vi "GUI - Text File (V1.00).vi"(0 "Time Data IN":refnum<class "GSwFormDSP.lvclass">, 5 "error in (no error)":errorcluster, 6 "Inlude Time Vector":bool, 7 "Application Name":string="GSwForm", 9 "State Queue":string[](array[string])=["SC: Initialize"], 11 "TextFile - READ":path, 13 "TextFile - WRITE":path) -> (14 "Time Data DUP":refnum<class "GSwFormDSP.lvclass">, 19 "error out":errorcluster)   [LabVIEW 2022 SP3, in "TEXT.lvclass"]
uses:
  TEXT.lvclass
  API/GSwFormDSP_class/GSwFormDSP.lvclass
  <vilib>/Utility/sysdir.llb/System Directory Type.ctl
  W:/projects/archives/23 Charette AI Group/SPWB/API/Generic Utilities_class/Generic Utilities.lvclass
  <vilib>/addons/_AddQ/G#Object/G#Object.lvclass
  API/Generic Utilities_class/Generic Utilities.lvclass
panel:
  in  "Task":enum32{"TDMS", "Settings"}(tab)
  out "Time Data":waveform(dbl)[](graph)
  in  "READ - Select Wave File":bool
  in  "WRITE - Select Wave File":bool
  out "State History":string[](array[string])
  out "State Index":i32
  in  "Exit":bool
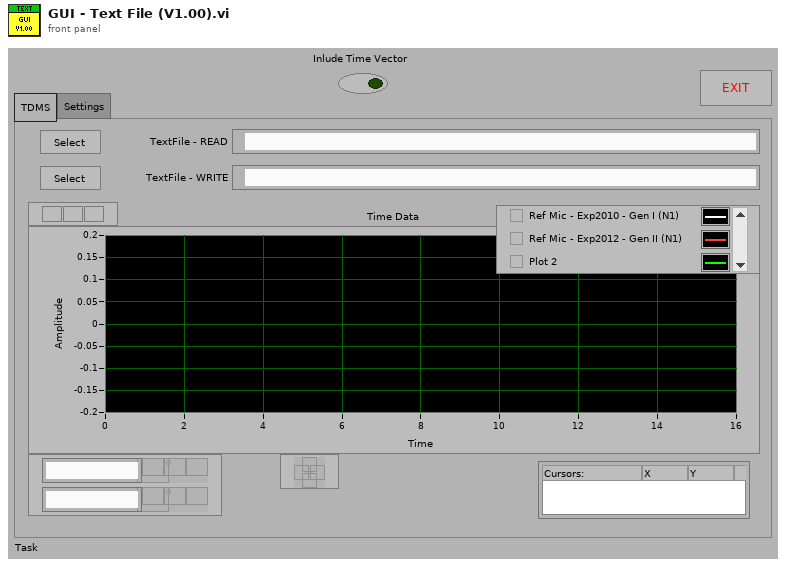
[diagram p1: front panel]
types:
  T1 = enum32{"Invalid", "Standard", "Closed", "Hidden", "Minimized", "Maximized"}
  T2 = typedef "System Directory Type.ctl" = i32
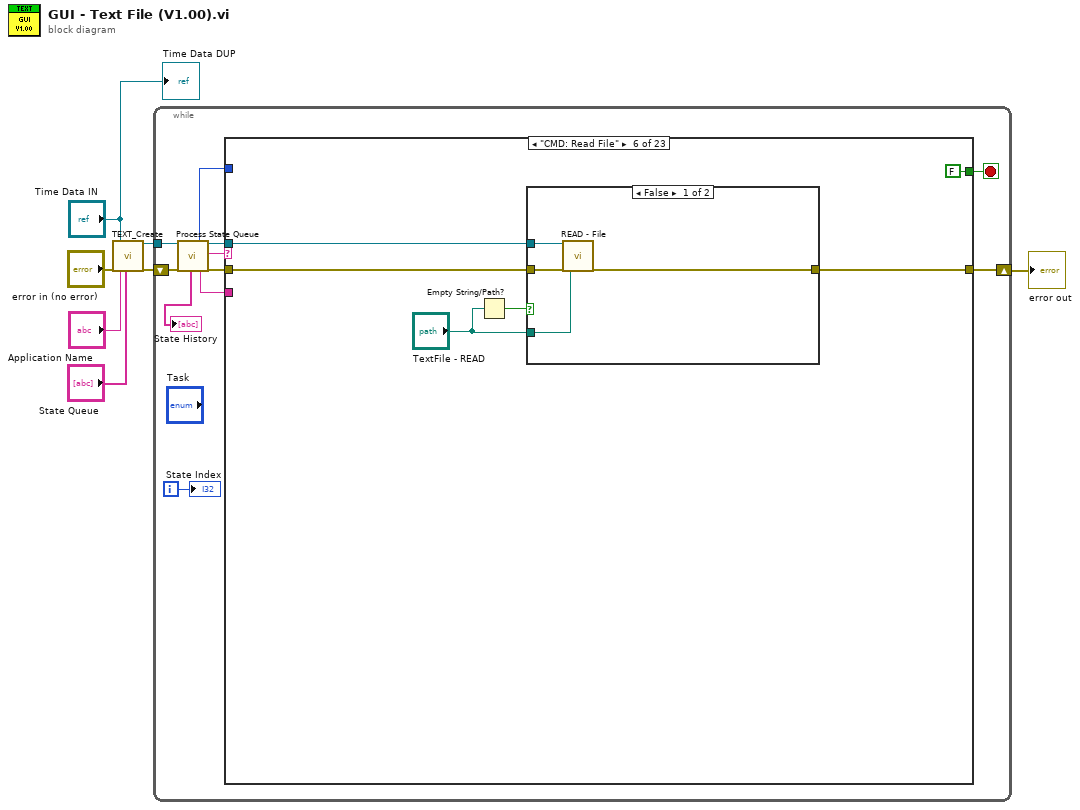
[diagram p0: block diagram]
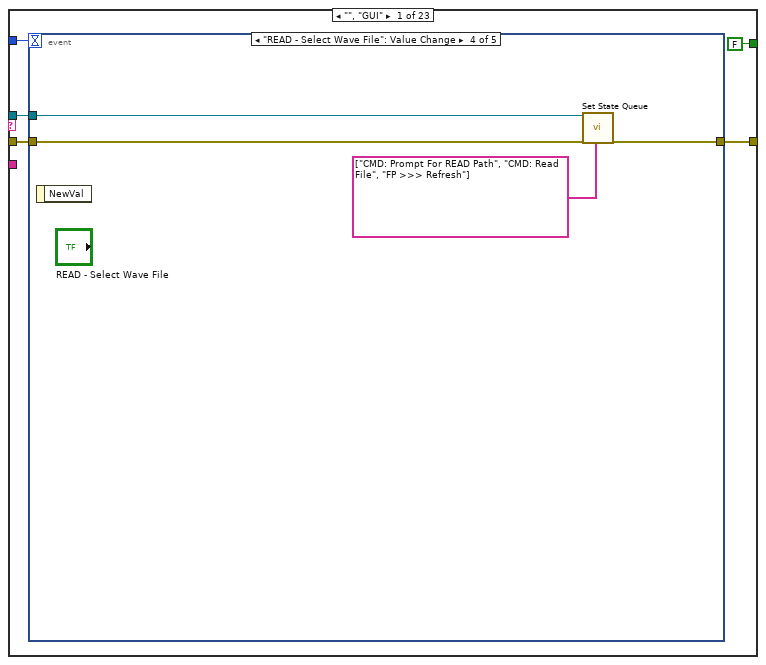
[diagram p2: hidden frame]
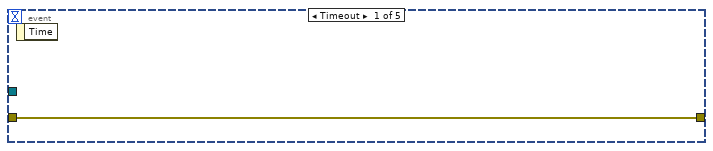
[diagram p3: hidden frame]
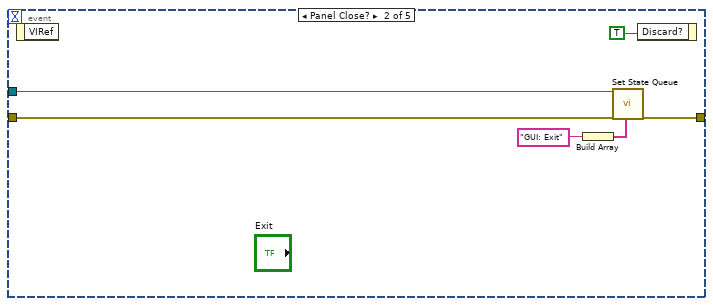
[diagram p4: hidden frame]
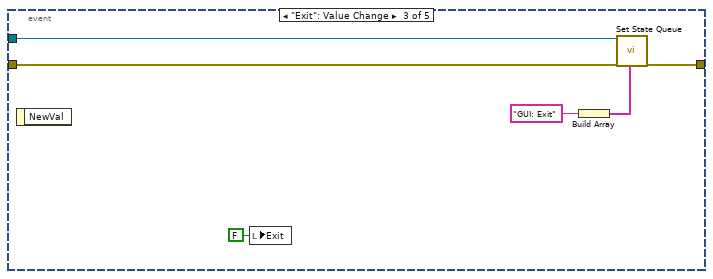
[diagram p5: hidden frame]
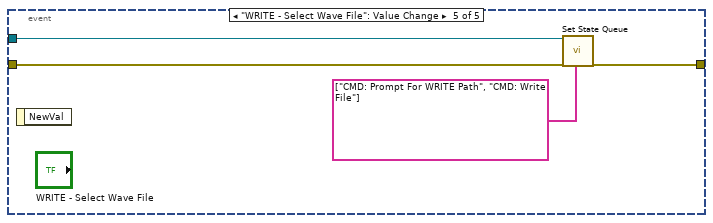
[diagram p6: hidden frame]
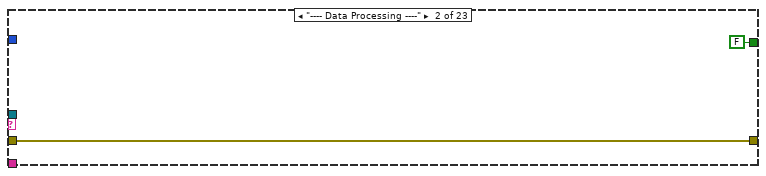
[diagram p7: hidden frame]
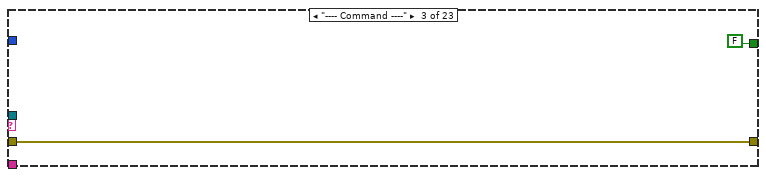
[diagram p8: hidden frame]
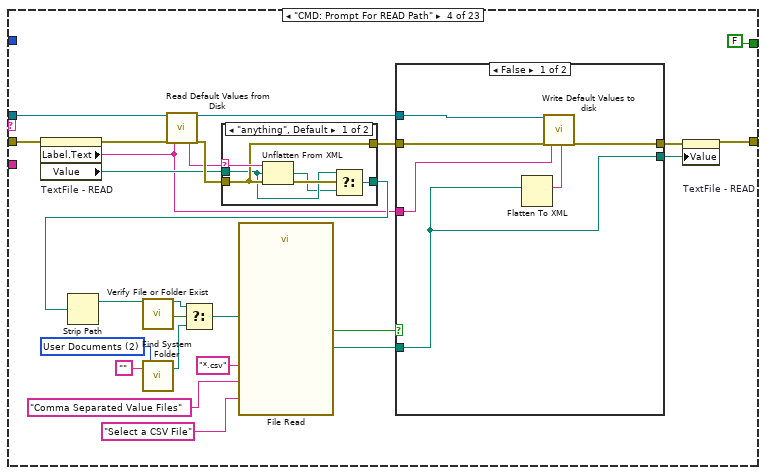
[diagram p9: hidden frame]
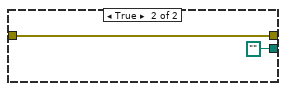
[diagram p10: hidden frame]
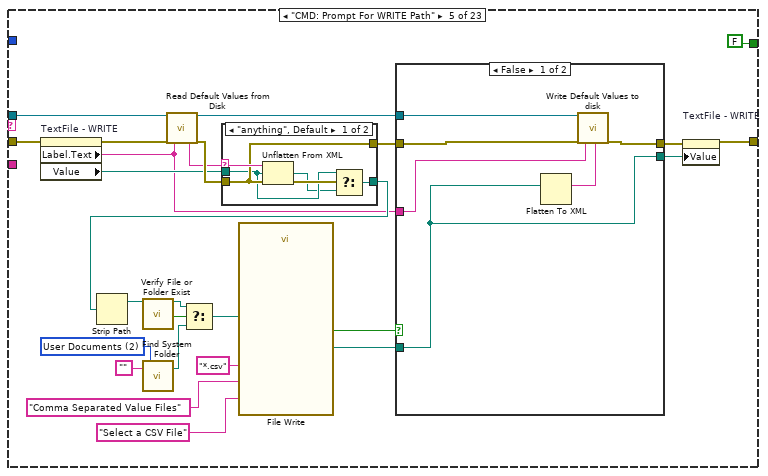
[diagram p12: hidden frame]
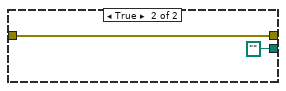
[diagram p13: hidden frame]
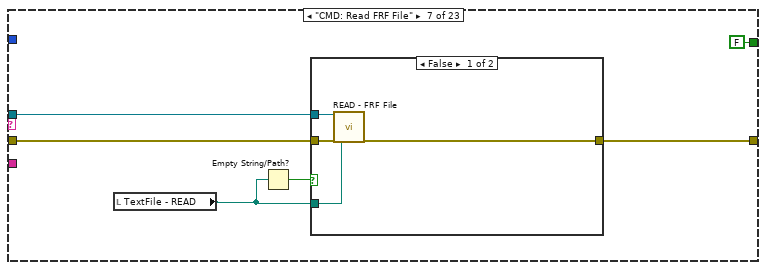
[diagram p16: hidden frame]
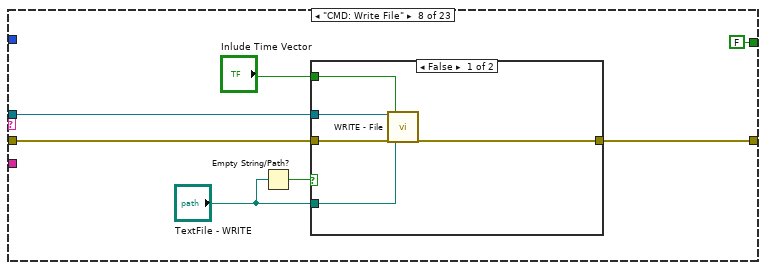
[diagram p18: hidden frame]
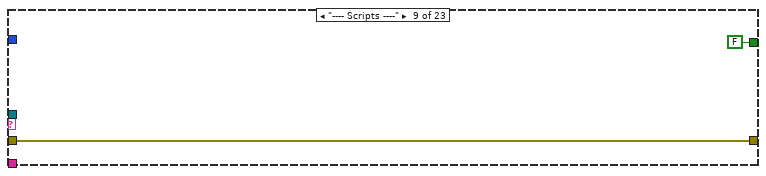
[diagram p20: hidden frame]
diagram:
  n1 = call "TEXT_Create.vi"("error in (no error)"="error in (no error)", "Time Data"="Time Data IN", "Application Name"="Application Name", "State Queue"="State Queue") -> ("reference out"=w7:refnum<class "TEXT.lvclass">, "error out"=w6:errorcluster)  [unwired: 14 in]
  n2 = while {
    shift-right: [w9] -> w2
    shift-left: w6 -> [w15]
    tunnel: w7 -> [w16]
    i -> [w17]
    stop <- w18 stop-if-true
    n3 = call "Process State Queue.vi"("reference in"=w16, "error in (no error)"=w15) -> ("State History"=→"State History":string[], "Timeout"=w14:i32, "State Option"=w11:string, "reference out"=w13:refnum<class "TEXT.lvclass">, "Current State"=w12:string, "error out"=w10:errorcluster)  [unwired: 10 in, 2 out]
    n4 = case shown="\"CMD: Read File\"" w12 {
      selector: w12 -> [_ _ _ _ _ _ _ _ _ _ _ _ _ _ _ _ _ _ _ w344 _ _ _]
      tunnel: w13 -> [w21 _ _ w73 w115 w137 w148 w160 _ w173 _ w179 w209 _ w249 w268 w301 w326 _ _ _ _ w352]
      tunnel: [FALSE FALSE FALSE FALSE FALSE FALSE FALSE FALSE FALSE FALSE FALSE FALSE FALSE FALSE FALSE TRUE FALSE FALSE FALSE FALSE FALSE FALSE TRUE] -> w18
      tunnel: w14 -> [w22 _ _ _ _ _ _ _ _ _ _ _ _ _ _ _ _ _ _ _ _ _ _]
      tunnel: w11 -> [_ _ _ _ _ _ _ _ _ _ _ w180 w206 _ _ _ w310 _ _ _ _ _ _]
      tunnel: w10 -> [w20 w45 w47 w72 w114 w136 w147 w159 w168 w172 w175 w177 w208 w235 w246 w265 w300 w327 w340 w342 w347 w350 w353]
      tunnel: [w19 w45 w47 w56 w100 w135 w146 w158 w168 w171 w175 w178 w207 w235 w237 w264 w298 w323 w340 w342 errorcluster {"status"=FALSE, "code"=0, "source"=""} ("error out") w350 w354] -> w9
      frame "", "GUI" {
        n5 = event shown="[3] \"READ - Select Wave File\": Value Change" {
          selector: _ -> [_ _ _ _ _]
          dyn-events: _ -> [_ _ _ _ _]
          timeout: w22 -> [_ _ _ _ _]
          tunnel: w21 -> [_ w28 w34 w39 w43]
          tunnel: w20 -> [w24 w27 w32 w38 w42]
          tunnel: [w24 w26 w33 w40 w44] -> w19
          event Timeout {
            n6 = event-data() -> ()  [unwired: 1 in, 1 out]
          }
          event Panel Close? {
            n7 = event-data() -> ()  [unwired: 1 in, 1 out]
            n8 = Build Array("GUI: Exit") -> (w25:string[])
            n9 = call "Set State Queue.vi"("reference in"=w28, "error in (no error)"=w27, "State Queue"=w25) -> ("error out"=w26:errorcluster)  [unwired: 15 in, 1 out]
            n10 = event-data("Discard?"=TRUE) -> ()  [unwired: 1 in, 1 out]
          }
          event "Exit": Value Change {
            n11 = event-data() -> ()  [unwired: 1 in, 1 out]
            n12 = local write "Exit"(FALSE ("Exit")) -> ()
            n13 = Build Array("GUI: Exit") -> (w31:string[])
            n14 = call "Set State Queue.vi"("reference in"=w34, "error in (no error)"=w32, "State Queue"=w31) -> ("error out"=w33:errorcluster)  [unwired: 15 in, 1 out]
          }
          event "READ - Select Wave File": Value Change {
            n15 = event-data() -> ()  [unwired: 1 in, 1 out]
            n16 = call "Set State Queue.vi"("reference in"=w39, "error in (no error)"=w38, "State Queue"=string[] ["CMD: Prompt For READ Path", "CMD: Read File", "FP >>> Refresh"]) -> ("error out"=w40:errorcluster)  [unwired: 15 in, 1 out]
          }
          event "WRITE - Select Wave File": Value Change {
            n17 = event-data() -> ()  [unwired: 1 in, 1 out]
            n18 = call "Set State Queue.vi"("reference in"=w43, "error in (no error)"=w42, "State Queue"=string[] ["CMD: Prompt For WRITE Path", "CMD: Write File"]) -> ("error out"=w44:errorcluster)  [unwired: 15 in, 1 out]
          }
        }
      }
      frame "---- Data Processing ----" {
      }
      frame "---- Command ----" {
      }
      frame "CMD: Prompt For READ Path" {
        w63 = T2 2 items=["User Home"=0, "User Desktop"=1, "User Documents"=2, "User Application Data"=3, "User Preferences"=4, "User Temporary"=5, "Public Documents"=6, "Public Application Data"=7, "Public Preferences"=8, "Public Cache"=13, "System Core Libraries"=9, "System Installed Libraries"=10, "Application Files"=11, "Boot Volume Root"=12] ("system directory type")
        n19 = property on="TextFile - READ" class="Path"(error in=w72) -> (error out=w71:errorcluster, "Label.Text"=w51:string, "Value"=w69:path)  [unwired: 1 in, 1 out]
        n20 = call "Find System Folder.vi"("Application Name"="", "system directory type"=w63) -> ("System Folder"=w62:path)  [unwired: 16 in, 1 out]
        n21 = call-dynamic "Read Default Values from Disk.vi"("reference in"=w73, "error in (no error)"=w71, "Control Label"=w51) -> ("Value (XML String)"=w49:string, "reference out"=w52:refnum<class "TEXT.lvclass">, "error out"=w70:errorcluster)  [unwired: 14 in]
        n22 = case shown="\"anything\", Default" w49 {
          selector: w49 -> [w88 _]
          tunnel: [w83 w90] -> w68
          tunnel: w69 -> [w85 w90]
          tunnel: w70 -> [w86 w89]
          tunnel: [w86 w89] -> w54
          frame "anything", Default {
            n23 = Unflatten From XML(xml string=w88, type=w85, error in (no error)=w86) -> (value=w84:path, error out=w87:errorcluster)
            n24 = Select(t=w85, s=w87, f=w84) -> (s? t:f=w83:path)
          }
          frame "" {
            # "Either the file was not found or there was some error"
          }
        }
        n25 = Strip Path(path=w68) -> (stripped path=w67:path)  [unwired: 1 out]
        n26 = call "Verify File or Folder Exist.vi"("path"=w67) -> ("dup path"=w65:path, "file or folder exists?"=w66:bool)  [unwired: 16 in, 1 out]
        n27 = Select(t=w65, s=w66, f=w62) -> (s? t:f=w64:path)
        n28 = call "File Read"("start path"=w64, "button label"="Select a CSV File", "pattern (all files)"="*.csv", "pattern label"="Comma Separated Value Files") -> ("selected path"=w50:path, "cancelled"=w57:bool)  [unwired: 8 in, 2 out]
        n29 = case shown="False" w57 {
          tunnel: [w76 w82] -> w55
          tunnel: w54 -> [w77 w82]
          tunnel: [w75 path ""] -> w53
          tunnel: w52 -> [w79 _]
          tunnel: w51 -> [w78 _]
          tunnel: w50 -> [w75 _]
          frame False {
            n30 = Flatten To XML(6:w75) -> (2:w80:string)
            n31 = call-dynamic "Write Default Values to disk.vi"("reference in"=w79, "error in (no error)"=w77, "Control Label"=w78, "Value (XML String)"=w80) -> ("error out"=w76:errorcluster)  [unwired: 14 in, 1 out]
          }
          frame True {
          }
        }
        n32 = property on="TextFile - READ" class="Path"(error in=w55, "Value"=w53) -> (error out=w56:errorcluster)  [unwired: 1 in, 1 out]
      }
      frame "CMD: Prompt For WRITE Path" {
        w105 = T2 2 items=["User Home"=0, "User Desktop"=1, "User Documents"=2, "User Application Data"=3, "User Preferences"=4, "User Temporary"=5, "Public Documents"=6, "Public Application Data"=7, "Public Preferences"=8, "Public Cache"=13, "System Core Libraries"=9, "System Installed Libraries"=10, "Application Files"=11, "Boot Volume Root"=12] ("system directory type")
        n33 = property on="TextFile - WRITE" class="Path"(error in=w114) -> (error out=w113:errorcluster, "Label.Text"=w95:string, "Value"=w111:path)  [unwired: 1 in, 1 out]
        n34 = call "Find System Folder.vi"("Application Name"="", "system directory type"=w105) -> ("System Folder"=w104:path)  [unwired: 16 in, 1 out]
        n35 = call-dynamic "Read Default Values from Disk.vi"("reference in"=w115, "error in (no error)"=w113, "Control Label"=w95) -> ("Value (XML String)"=w91:string, "reference out"=w96:refnum<class "TEXT.lvclass">, "error out"=w112:errorcluster)  [unwired: 14 in]
        n36 = case shown="\"anything\", Default" w91 {
          selector: w91 -> [w130 _]
          tunnel: [w125 w132] -> w110
          tunnel: w111 -> [w127 w132]
          tunnel: w112 -> [w128 w131]
          tunnel: [w128 w131] -> w98
          frame "anything", Default {
            n37 = Unflatten From XML(xml string=w130, type=w127, error in (no error)=w128) -> (value=w126:path, error out=w129:errorcluster)
            n38 = Select(t=w127, s=w129, f=w126) -> (s? t:f=w125:path)
          }
          frame "" {
            # "Either the file was not found or there was some error"
          }
        }
        n39 = Strip Path(path=w110) -> (stripped path=w109:path)  [unwired: 1 out]
        n40 = call "Verify File or Folder Exist.vi"("path"=w109) -> ("dup path"=w107:path, "file or folder exists?"=w108:bool)  [unwired: 16 in, 1 out]
        n41 = Select(t=w107, s=w108, f=w104) -> (s? t:f=w106:path)
        n42 = call "File Write"("start path"=w106, "button label"="Select a CSV File", "pattern (all files)"="*.csv", "pattern label"="Comma Separated Value Files") -> ("selected path"=w94:path, "cancelled"=w101:bool)  [unwired: 8 in, 2 out]
        n43 = case shown="False" w101 {
          tunnel: [w118 w124] -> w99
          tunnel: w98 -> [w119 w124]
          tunnel: [w117 path ""] -> w97
          tunnel: w96 -> [w121 _]
          tunnel: w95 -> [w120 _]
          tunnel: w94 -> [w117 _]
          frame False {
            n44 = Flatten To XML(6:w117) -> (2:w122:string)
            n45 = call-dynamic "Write Default Values to disk.vi"("reference in"=w121, "error in (no error)"=w119, "Control Label"=w120, "Value (XML String)"=w122) -> ("error out"=w118:errorcluster)  [unwired: 14 in, 1 out]
          }
          frame True {
          }
        }
        n46 = property on="TextFile - WRITE" class="Path"(error in=w99, "Value"=w97) -> (error out=w100:errorcluster)  [unwired: 1 in, 1 out]
      }
      frame "CMD: Read File" {
        n47 = Empty String/Path?(string/path="TextFile - READ") -> (empty?=w134:bool)
        n48 = case shown="False" w134 {
          tunnel: w137 -> [w142 _]
          tunnel: w136 -> [w141 w143]
          tunnel: [w139 w143] -> w135
          tunnel: "TextFile - READ" -> [w140 _]
          frame False {
            n49 = call "READ - File.vi"("reference in"=w142, "error in (no error)"=w141, "TDMS Path - READ"=w140) -> ("error out"=w139:errorcluster)  [unwired: 15 in, 1 out]
          }
          frame True {
            # "User cancelled, so do nothing!"
          }
        }
      }
      frame "CMD: Read FRF File" {
        n50 = local read "TextFile - READ"() -> (w144:path)
        n51 = Empty String/Path?(string/path=w144) -> (empty?=w145:bool)
        n52 = case shown="False" w145 {
          tunnel: w148 -> [w153 _]
          tunnel: w147 -> [w152 w154]
          tunnel: [w150 w154] -> w146
          tunnel: w144 -> [w151 _]
          frame False {
            n53 = call "READ - FRF File.vi"("reference in"=w153, "error in (no error)"=w152, "TDMS Path - READ"=w151) -> ("error out"=w150:errorcluster)  [unwired: 15 in, 1 out]
          }
          frame True {
            # "User cancelled, so do nothing!"
          }
        }
      }
      frame "CMD: Write File" {
        n54 = Empty String/Path?(string/path="TextFile - WRITE") -> (empty?=w157:bool)
        n55 = case shown="False" w157 {
          tunnel: w160 -> [w166 _]
          tunnel: w159 -> [w165 w167]
          tunnel: [w163 w167] -> w158
          tunnel: "TextFile - WRITE" -> [w164 _]
          tunnel: "Inlude Time Vector" -> [w162 _]
          frame False {
            n56 = call "WRITE - File.vi"("reference in"=w166, "error in (no error)"=w165, "Inlude Time Vector"=w162, "CSV Path - WRITE"=w164) -> ("error out"=w163:errorcluster)  [unwired: 14 in, 1 out]
          }
          frame True {
            # "User cancelled, so do nothing!"
          }
        }
      }
      frame "---- Scripts ----" {
      }
      frame "SC: Initialize" {
        n57 = call "Set State Queue.vi"("reference in"=w173, "error in (no error)"=w172, "State Queue"=string[] ["GUI: Initialize Ref", "FP >>> Open"] ("State Queue OUT")) -> ("error out"=w171:errorcluster)  [unwired: 15 in, 1 out]
      }
      frame "---- Front Panel Mgmt ----" {
      }
      frame "CTRL" {
        n58 = case shown="\"Task Tab\"" w180 {
          selector: w180 -> [w185 _]
          tunnel: [w183 w190] -> _
          tunnel: w179 -> [w183 w195]
          tunnel: [w182 w189] -> w178
          tunnel: w177 -> [w182 w193]
          frame "unknown", Default {
            n59 = Concatenate Strings("The following control name is unrecognized:\n", w185) -> (w184:string)
            n60 = One Button Dialog(message=w184) -> ()  [unwired: 1 in, 1 out]
          }
          frame "Task Tab" {
            n61 = property on="TextFile - READ" class="Path"(error in=w193) -> (error out=w194:errorcluster, "Label.Text"=w192:string, "Value"=w197:path)  [unwired: 1 in, 1 out]
            n62 = call-dynamic "Read Default Values from Disk.vi"("reference in"=w195, "error in (no error)"=w194, "Control Label"=w192) -> ("Value (XML String)"=w187:string, "reference out"=w190:refnum<class "TEXT.lvclass">, "error out"=w191:errorcluster)  [unwired: 14 in]
            n63 = case shown="\"anything\", Default" w187 {
              selector: w187 -> [w203 _]
              tunnel: [w198 w205] -> w188
              tunnel: w197 -> [w200 w205]
              tunnel: w191 -> [w201 w204]
              tunnel: [w201 w204] -> w196
              frame "anything", Default {
                n64 = Unflatten From XML(xml string=w203, type=w200, error in (no error)=w201) -> (value=w199:path, error out=w202:errorcluster)
                n65 = Select(t=w200, s=w202, f=w199) -> (s? t:f=w198:path)
              }
              frame "" {
                # "Either the file was not found or there was some error"
              }
            }
            n66 = property on="TextFile - READ" class="Path"(error in=w196, "Value"=w188) -> (error out=w189:errorcluster)  [unwired: 1 in, 1 out]
          }
        }
      }
      frame "FP" {
        n67 = case shown="\"Refresh\"" w206 {
          selector: w206 -> [w212 _ _]
          tunnel: w209 -> [_ w219 w232]
          tunnel: w208 -> [w211 w218 w231]
          tunnel: [w211 w215 w229] -> w207
          frame "", Default {
            n68 = Concatenate Strings("The following FP is unrecognized:\n", w212) -> (w213:string)
            n69 = One Button Dialog(message=w213) -> ()  [unwired: 1 in, 1 out]
          }
          frame "Open" {
            n70 = call-dynamic "Get VI Ref.vi"("reference in"=w219, "error in (no error)"=w218) -> ("GUI VI Ref"=w216:refnum<vi>, "error out"=w217:errorcluster)  [unwired: 14 in, 2 out]
            n71 = property class="VI"(reference=w216, error in=w217) -> (reference out=w221:refnum<vi>, error out=w222:errorcluster, "Front Panel.Open"=w220:bool)
            n72 = case shown="False" w220 {
              tunnel: [w225 w228] -> w215
              tunnel: w222 -> [w224 w228]
              tunnel: w221 -> [w223 _]
              frame False {
                n73 = invoke class="VI" method="FP.Open"(reference=w223, error in=w224, "Activate"=TRUE, "State"=T1."Standard") -> (error out=w225:errorcluster)  [unwired: 1 in, 4 out]
              }
              frame True {
              }
            }
          }
          frame "Refresh" {
            n74 = call "Get - Time Data OBJ.vi"("reference in"=w232, "error in (no error)"=w231) -> ("Time Data OBJ"=w234:refnum<class "GSwFormDSP.lvclass">, "error out"=w233:errorcluster)  [unwired: 15 in, 1 out]
            n75 = call-dynamic "Get - wForms.vi"("reference in"=w234, "error in (no error)"=w233) -> ("wForms"=→"Time Data":waveform(dbl)[], "error out"=w229:errorcluster)  [unwired: 14 in, 2 out]
          }
        }
      }
      frame "---- GUI Functions ----" {
      }
      frame "GUI: Initialize Ref" {
        n76 = control-ref of="GUI Reference"() -> (w245:refnum<vi>)
        n77 = call "Set VI Ref.vi"("reference in"=w249, "error in (no error)"=w246, "GUI VI Ref"=w245) -> ("reference out"=w248:refnum<class "TEXT.lvclass">, "error out"=w244:errorcluster)  [unwired: 15 in]
        n78 = call "Set Close Panel (Yes or No).vi"("reference in"=w248, "error in (no error)"=w244) -> ("reference out"=w247:refnum<class "TEXT.lvclass">, "error out"=w243:errorcluster)  [unwired: 16 in]
        n79 = call "Set Message Window Ref.vi"("reference in"=w247, "error in (no error)"=w243) -> ("reference out"=w241:refnum<class "TEXT.lvclass">, "error out"=w242:errorcluster)  [unwired: 16 in]
        n80 = call "Get - Time Data OBJ State.vi"("reference in"=w241, "error in (no error)"=w242) -> ("New Time Data Obj?"=w240:bool, "reference out"=w239:refnum<class "TEXT.lvclass">, "error out"=w238:errorcluster)  [unwired: 15 in]
        n81 = case shown="True" w240 {
          tunnel: w239 -> [_ w257]
          tunnel: w238 -> [w251 w256]
          tunnel: [w251 w252] -> w237
          frame False {
          }
          frame True {
            n82 = call "Get - Time Data OBJ.vi"("reference in"=w257, "error in (no error)"=w256) -> ("Time Data OBJ"=w254:refnum<class "GSwFormDSP.lvclass">, "error out"=w253:errorcluster)  [unwired: 15 in, 1 out]
            n83 = call "Set - wForms.vi"("reference in"=w254, "error in (no error)"=w253, "Init wForms"=TRUE) -> ("error out"=w252:errorcluster)  [unwired: 15 in, 1 out]
          }
        }
      }
      frame "GUI: Exit" {
        n84 = call-dynamic "Get Message Window Ref.vi"("reference in"=w268, "error in (no error)"=w265) -> ("reference out"=w267:refnum<class "TEXT.lvclass">, "Msg Win Ref"=w263:refnum<vi>, "error out"=w266:errorcluster)  [unwired: 15 in]
        n85 = call-dynamic "Get VI Ref.vi"("reference in"=w267, "error in (no error)"=w266) -> ("reference out"=w272:refnum<class "TEXT.lvclass">, "GUI VI Ref"=w270:refnum<vi>, "error out"=w271:errorcluster)  [unwired: 14 in, 1 out]
        n86 = call-dynamic "Get Close Panel (Yes or No).vi"("reference in"=w272, "error in (no error)"=w271) -> ("Close Panel?"=w273:bool, "reference out"=w262:refnum<class "TEXT.lvclass">, "error out"=w260:errorcluster)  [unwired: 15 in]
        n87 = call "Get - Time Data OBJ State.vi"("reference in"=w262, "error in (no error)"=w260) -> ("New Time Data Obj?"=w258:bool, "reference out"=w261:refnum<class "TEXT.lvclass">, "error out"=w259:errorcluster)  [unwired: 15 in]
        n88 = call-dynamic "Destroy.vi"("reference in"=w261, "error in (no error)"=w259) -> ("error out"=w277:errorcluster)  [unwired: 16 in, 1 out]
        n89 = case shown="True" w258 {
          tunnel: w277 -> [w279 w281]
          tunnel: [w279 w280] -> w269
          frame False {
          }
          frame True {
            n90 = call <vilib>:"GarbageCollector.vi"("error in (no error)"=w281) -> ("error out"=w280:errorcluster)  [unwired: 16 in, 2 out]
          }
        }
        n91 = Close Reference(reference=w263, error in (no error)=w269) -> (error out=w276:errorcluster)
        n92 = case shown="True" w273 {
          tunnel: w276 -> [w283 w287]
          tunnel: [w283 w286] -> w274
          tunnel: [w282 w285] -> w275
          tunnel: w270 -> [w282 w284]
          frame False {
          }
          frame True {
            n93 = property class="VI"(reference=w284, error in=w287) -> (reference out=w289:refnum<vi>, error out=w288:errorcluster, "Front Panel.Open"=w290:bool)
            n94 = case shown="True" w290 {
              tunnel: [w292 w296] -> w286
              tunnel: w288 -> [w292 w295]
              tunnel: w289 -> [w291 w294]
              tunnel: [w291 w293] -> w285
              frame False {
              }
              frame True {
                n95 = invoke class="VI" method="FP.Close"(reference=w294, error in=w295) -> (reference out=w293:refnum<vi>, error out=w296:errorcluster)  [unwired: 1 in, 1 out]
              }
            }
          }
        }
        n96 = Close Reference(reference=w275, error in (no error)=w274) -> (error out=w264:errorcluster)
      }
      frame "SEND MSG" {
        n97 = call-dynamic "Get Message Window Ref.vi"("reference in"=w301, "error in (no error)"=w300) -> ("Msg Win Ref"=w297:refnum<vi>, "error out"=w299:errorcluster)  [unwired: 15 in, 1 out]
        n98 = property class="VI"(reference=w297, error in=w299) -> (reference out=w303:refnum<vi>, error out=w302:errorcluster, "Front Panel.Open"=w304:bool)
        n99 = case shown="False" w304 {
          tunnel: [w318 w322] -> w306
          tunnel: w302 -> [w313 w322]
          tunnel: w303 -> [w315 w321]
          tunnel: [w317 w321] -> w305
          frame False {
            w316 = FALSE ("Wait Until Done")
            n100 = invoke class="VI" method="Run VI"(reference=w315, error in=w313, "Wait until done"=w316, "Auto Dispose Ref"=w316) -> (reference out=w314:refnum<vi>, error out=w312:errorcluster)  [unwired: 1 in, 3 out]
            n101 = invoke class="VI" method="FP.Open"(reference=w314, error in=w312, "Activate"=TRUE, "State"=T1."Standard") -> (reference out=w317:refnum<vi>, error out=w318:errorcluster)  [unwired: 1 in, 3 out]
          }
          frame True {
          }
        }
        n102 = Concatenate Strings("\r\n", w310) -> (w309:string)
        n103 = invoke class="VI" method="Ctrl Val.Set"(reference=w305, error in=w306, "Control Name"="Message", "Value"=w309) -> (error out=w298:errorcluster)  [unwired: 1 in, 4 out]
      }
      frame "CLOSE MSG" {
        n104 = call-dynamic "Get Message Window Ref.vi"("reference in"=w326, "error in (no error)"=w327) -> ("Msg Win Ref"=w324:refnum<vi>, "error out"=w325:errorcluster)  [unwired: 15 in, 1 out]
        n105 = property class="VI"(reference=w324, error in=w325) -> (reference out=w331:refnum<vi>, error out=w332:errorcluster, "Front Panel.Open"=w330:bool)
        n106 = case shown="True" w330 {
          tunnel: [w335 w339] -> w329
          tunnel: w332 -> [w335 w338]
          tunnel: w331 -> [w334 w337]
          tunnel: [w334 w336] -> w328
          frame False {
          }
          frame True {
            n107 = invoke class="VI" method="FP.Close"(reference=w337, error in=w338) -> (reference out=w336:refnum<vi>, error out=w339:errorcluster)  [unwired: 1 in, 1 out]
          }
        }
        n108 = invoke class="VI" method="Abort VI"(reference=w328, error in=w329) -> (error out=w323:errorcluster)  [unwired: 1 in, 2 out]
      }
      frame "---- Miscelleneous ----" {
      }
      frame "unknown", Default {
        n109 = Concatenate Strings("The following state is unrecognized?\n", w344) -> (w343:string)
        n110 = One Button Dialog(message=w343) -> ()  [unwired: 1 in, 1 out]
      }
      frame "Error" {
        n111 = call <vilib>:"General Error Handler.vi"("error in (no error)"=w347) -> ()  [unwired: 10 in, 5 out]
      }
      frame "Next" {
        # "This is an empty case used so the queue does NOT stop if there is an empty string between two valid states!"
      }
      frame "Quit" {
        # "This is the case used to simply exit when this GUI is used as a SubVI!"
        n112 = call-dynamic "Destroy.vi"("reference in"=w352, "error in (no error)"=w353) -> ("error out"=w354:errorcluster)  [unwired: 16 in, 1 out]
      }
    }
    "State Index" <- w17
  }
  "error out" <- w2
  "Time Data DUP" <- "Time Data IN"
